vi "initScale.vi"(8 "error in (no error)":errorcluster, 11 "OHAUS AV8101 in":refnum<class "OHAUS AV8101.lvclass">) -> (0 "error out":errorcluster, 3 "OHAUS AV8101 out":refnum<class "OHAUS AV8101.lvclass">)   [LabVIEW 2015, in "OHAUS AV8101.lvclass"]
uses:
  OHAUS AV8101.lvclass
  OHAUS AV8101.lvclass/OHAUS AV8101.ctl
  OHAUS AV8101 Drivers/Ohaus AV Series.lvlib
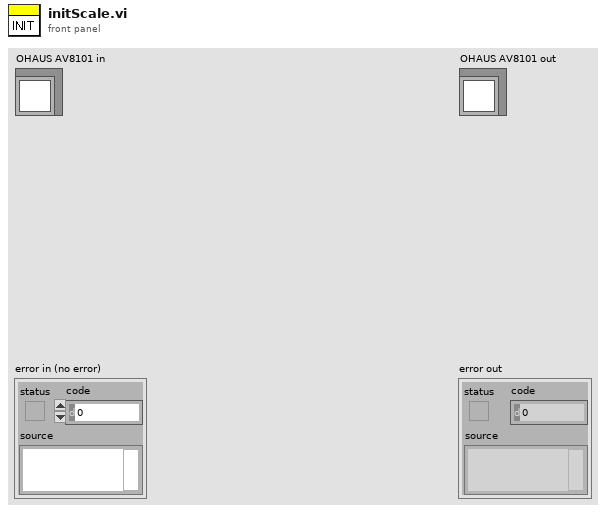
[diagram p1: front panel]
types:
  T1 = cluster{"Baud Rate (2400)":u32, "Flow Control (1: XON/XOFF)":u16, "Parity (0: None)":u16, "Data Bits (7)":u16}
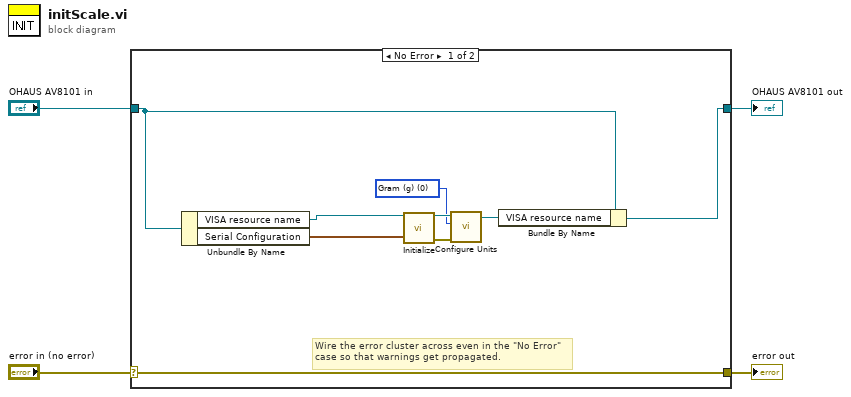
[diagram p0: block diagram]
diagram:
  n1 = case shown="No Error" "error in (no error)" {
    selector: "error in (no error)" -> [w13 w15]
    tunnel: [w13 w15] -> w3
    tunnel: [w5 w14] -> w1
    tunnel: "OHAUS AV8101 in" -> [w7 w14]
    frame No Error {
      w10 = u16 0 items=["Gram (g)"=0, "Kilogram (kg)"=1, "Penny weight (dwt)"=2, "Carat (ct)"=3, "Ounce (oz)"=4, "Ounce Troy (oz t)"=5, "Grain (GN)"=6, "Hong Kong Tael (HKt)"=7, "Singapore Tael (SGt)"=8, "Tiwan Tael (TWt)"=9, "Momme (m)"=10, "Pound (lb)"=11, "Newton (N)"=13, "Tical (ti)"=14, "Tula"=15, "Mesghal (Meshg)"=16, "Baht"=17, "Custom"=19] ("Units (0: Gram)")
      # "Wire the error cluster across even in the \"No Error\"\ncase so that warnings get propagated."
      n2 = Unbundle By Name(w7) -> ("VISA resource name"=w9:refnum<visa-resource-name>, "Serial Configuration"=w8:T1)
      n3 = call "Initialize.vi"("VISA resource name"=w9, "Serial Configuration"=w8) -> ("VISA resource name out"=w12:refnum<visa-resource-name>, "error out"=w11:errorcluster)  [unwired: 12 in]
      n4 = call "Configure Units.vi"("error in (no error)"=w11, "Units (0: Gram)"=w10, "VISA resource name"=w12) -> ("VISA resource name out"=w6:refnum<visa-resource-name>)  [unwired: 7 in, 1 out]
      n5 = Bundle By Name(cluster=w7, "VISA resource name"=w6) -> (w5:refnum<class "OHAUS AV8101.lvclass">)
    }
    frame Error {
    }
  }
  "error out" <- w3
  "OHAUS AV8101 out" <- w1
